vi "Validate WiFi Connection.vi"(7 "Retry wait time [ms]":u32=500, 8 "Error In":errorcluster, 10 "TCP Configuration":T5, 11 "LINX Resource":T1) -> (0 "error out":errorcluster, 1 "Connected?":bool, 2 "TCP Config out":T5, 3 "LINX Resource Out":T1)   [LabVIEW 2019, in "LINXx.lvlib"]
doc: "Verify that specified address matches that in board's memory. For DHCP, attempts to reset TCP connection and returns when a valid address is produced."
uses:
  LINXx.lvlib
  <vilib>/MakerHub/LINX/Private/Device/Type Defs/TCP Config.ctl
  <vilib>/MakerHub/LINX/Private/Type Defs/LINX Ref.ctl
  <vilib>/MakerHub/LINX/Private/Type Defs/Platform.ctl
  <vilib>/MakerHub/LINX/Private/Type Defs/Interface.ctl
  <vilib>/MakerHub/LINX/Private/Device/Type Defs/LINX Device Config.ctl
  <vilib>/MakerHub/LINX/Private/Device/Type Defs/Channels.ctl
  <vilib>/Utility/error.llb/DialogType.ctl
  <vilib>/MakerHub/LINX/Private/Device/Device.lvlib
  <vilib>/MakerHub/LINX/LMH-LINX.lvlib
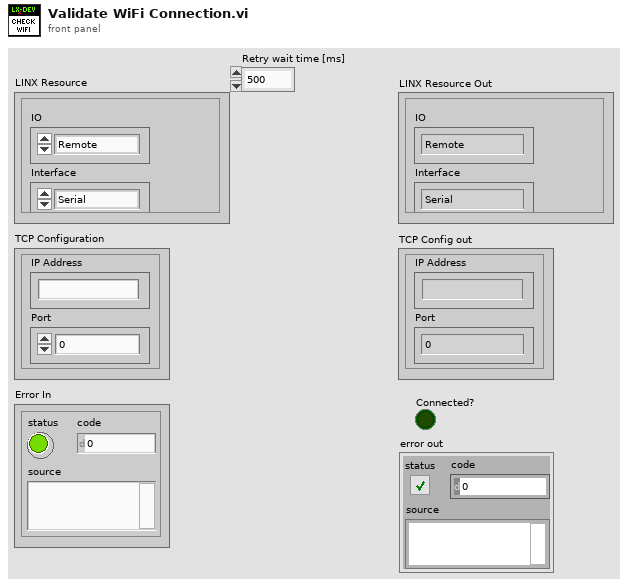
[diagram p1: front panel]
types:
  T1 = typedef "LMH-LINX.lvlib/LINX Ref.ctl" = cluster{"IO":T2, "Interface":T3, "LINX Device Config":T4}
  T2 = typedef "LMH-LINX.lvlib/Platform.ctl" = enum16{"Remote", "Local"}
  T3 = typedef "LMH-LINX.lvlib/Interface.ctl" = enum16{"Serial", "TCP"}
  T4 = typedef "LMH-LINX.lvlib/Device.lvlib/LINX Device Config.ctl" = cluster{"Interface":T3, "COM Port":refnum<visa-resource-name>, "TCP Configuration":T5, "Device Family":u8, "Device ID":u8, "Device Name":string, "TCP Ref":refnum<k5>, "Channels":T6}
  T5 = typedef "LMH-LINX.lvlib/Device.lvlib/TCP Config.ctl" = cluster{"IP Address":string, "Port":u16}
  T6 = typedef "LMH-LINX.lvlib/Channels.ctl" = cluster{"DI":u8[], "DO":u8[], "AI":u8[], "AO":u8[], "PWM":u8[], "QE":u8[], "UART":u8[], "I2C 2":u8[], "SPI":u8[], "CAN":u8[], "Servo":u8[], "AI Ref (V)":dbl, "AI Resolution (Bits)":u8, "AO Ref (V)":dbl, "AO Resolution (Bits)":u8}
  T7 = typedef "DialogType.ctl" = u16
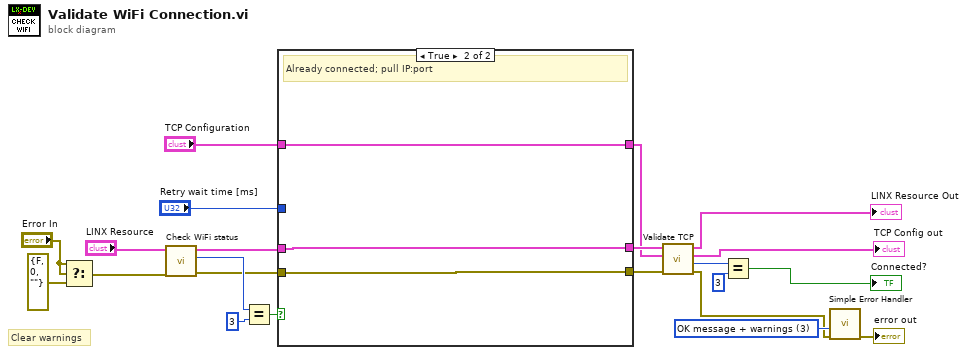
[diagram p0: block diagram]
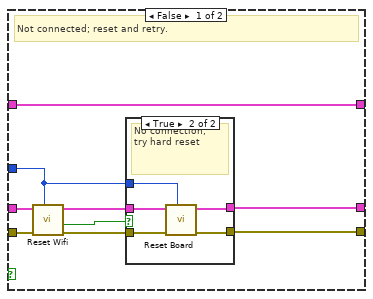
[diagram p2: hidden frame]
diagram:
  w22 = T7 3 items=["no dialog", "OK message", "continue or stop message", "OK message + warnings", "continue/stop + warnings"] ("type of dialog (OK msg:1)")
  # "Clear warnings"
  n1 = Select(t="Error In", s="Error In", f=errorcluster {"status"=FALSE, "code"=0, "source"=""}) -> (s? t:f=w5:errorcluster)
  n2 = call "Check WiFi status.vi"("Error In"=w5, "LINX Resource"="LINX Resource") -> ("Error Out"=w2:errorcluster, "WiFi status"=w3:u8, "LINX Resource out"=w4:T1)  [unwired: 7 in]
  n3 = Equal?(x=w3, y=u8 3) -> (x = y?=w20:bool)
  n4 = case shown="True" w20 {
    tunnel: w2 -> [w30 w40]
    tunnel: w4 -> [w31 w41]
    tunnel: "Retry wait time [ms]" -> [w28 _]
    tunnel: [w25 w40] -> w13
    tunnel: [w24 w41] -> w12
    tunnel: [w23 w39] -> w1
    tunnel: "TCP Configuration" -> [w23 w39]
    frame False {
      # "Not connected; reset and retry."
      n5 = call "Reset Wifi.vi"("Retry wait time [ms]"=w28, "error in (no error)"=w30, "LINX Resource"=w31) -> ("error out"=w26:errorcluster, "Connected to network?"=w29:bool, "LINX Resource Out"=w27:T1)  [unwired: 5 in, 1 out]
      n6 = case shown="True" w29 {
        tunnel: w28 -> [_ w34]
        tunnel: w27 -> [w32 w38]
        tunnel: [w32 w35] -> w24
        tunnel: w26 -> [w33 w37]
        tunnel: [w33 w36] -> w25
        frame False {
        }
        frame True {
          # "No connection;\ntry hard reset"
          n7 = call "Reset Board.vi"("Reconnect wait time"=w34, "Error In"=w37, "LINX Resource"=w38) -> ("Error Out"=w36:errorcluster, "LINX Resource out"=w35:T1)  [unwired: 7 in]
        }
      }
    }
    frame True {
      # "Already connected; pull IP:port"
    }
  }
  n8 = call "Validate TCP.vi"("error in (no error)"=w13, "User TCP Configuration"=w1, "LINX Resource"=w12) -> ("error out"=w11:errorcluster, "WiFi status"=w10:u8, "Board TCP Configuration"=→"TCP Config out":T5, "LINX Resource Out"=→"LINX Resource Out":T1)  [unwired: 5 in]
  n9 = Equal?(x=w10, y=u8 3) -> (x = y?=→"Connected?":bool)
  n10 = call <vilib>:"Simple Error Handler.vi"("type of dialog (OK msg:1)"=w22, "error in (no error)"=w11) -> ("error out"=→"error out":errorcluster)  [unwired: 3 in, 4 out]
